vi "FisherPaykel Bridge Profile.vi"(7 "Debug":bool, 8 "Error In":errorcluster, 9 "Move with Bridge Test Profile":T1, 10 "Main Command":T2=">GB", 11 "VISA Refnum in":refnum<visa-resource-name>) -> (0 "Error Out":errorcluster, 2 "Command (Debug)":string, 3 "VISA Refnum out":refnum<visa-resource-name>)   [LabVIEW 2016]
uses:
  Type Definitions/Fisher Paykel Main Command.ctl
  Type Definitions/Fisher Paykel Bridge Test Profile.ctl
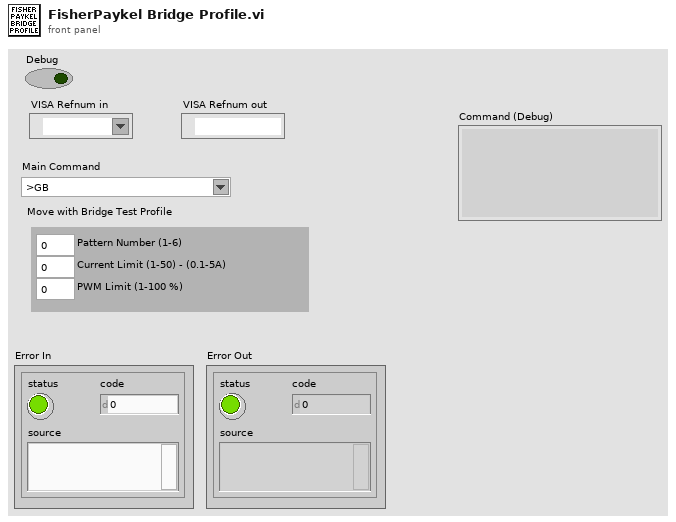
[diagram p1: front panel]
types:
  T1 = typedef "Fisher Paykel Bridge Test Profile.ctl" = cluster{"Pattern Number (1-6)":u16, "Current Limit (1-50) - (0.1-5A)":u16, "PWM Limit (1-100 %)":u16}
  T2 = typedef "Fisher Paykel Main Command.ctl" = string
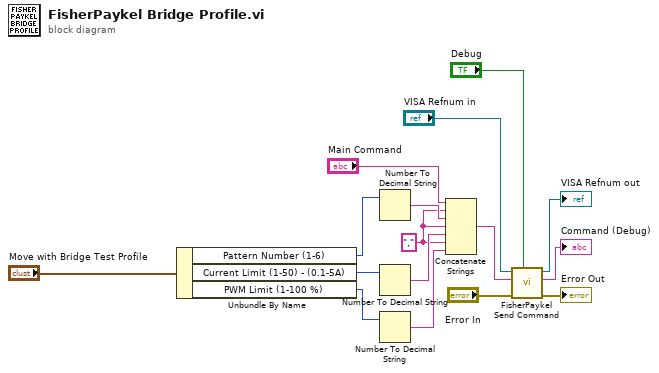
[diagram p0: block diagram]
diagram:
  w2 = ","
  n1 = Unbundle By Name("Move with Bridge Test Profile") -> ("Pattern Number (1-6)"=w8:u16, "Current Limit (1-50) - (0.1-5A)"=w7:u16, "PWM Limit (1-100 %)"=w3:u16)
  n2 = Number To Decimal String(number=w8) -> (decimal integer string=w6:string)  [unwired: 1 in]
  n3 = Number To Decimal String(number=w7) -> (decimal integer string=w5:string)  [unwired: 1 in]
  n4 = Number To Decimal String(number=w3) -> (decimal integer string=w1:string)  [unwired: 1 in]
  n5 = Concatenate Strings("Main Command", w2, w6, w2, w5, w2, w1) -> (w15:string)
  n6 = call "FisherPaykel Send Command.vi"("Debug"="Debug", "error in (no error)"="Error In", "Send Command"=w15, "VISA Refnum in"="VISA Refnum in") -> ("error out"=→"Error Out":errorcluster, "Command (Debug)"=→"Command (Debug)":string, "VISA Refnum out"=→"VISA Refnum out":refnum<visa-resource-name>)  [unwired: 5 in]
